vi "SparkFun Motor Driver.vi"() -> ()   [LabVIEW 2016]
uses:
  VIs/uPythonX/uPythonX.xctl
panel:
  in  "Tab Control":T1(tab)=enum."Tacho - interrupt"
  in  "Motors":T2(xcontrol)={"VISA Refnum in"="ASRL23::INSTR", "Python Code"="# In 1    In2    PWM   Out1    Out2    Mode\n#   H       H       H/L       L          L        short break\n#   L        H         H        L          H        CCW\n#   L        H         L        L          H        short break\n#   H        L         H       H          L        CW\n#   H        L         L        L          H       short break\n#   L         L         L        L          L        Stop\n\n# STBY must be high\n\nfrom pyb import Pin, Timer\n\nA_PWM = Pin('W29') # W29 has TIM2, CH2\nAIn2 = Pin('W22', Pin.OUT)\nAIn1 = Pin('W16',Pin.OUT)\nStdby = Pin('W24',Pin.OUT)\n\nBIn1 = Pin('Y12', Pin.OUT)\nBIn2 = Pin('W32',Pin.OUT)\nB_PWM = Pin('Y11') #  TIM8, CH2\n\ntimA = Timer(2, freq=1000)\ntimB = Timer(8, freq=1000)\n\nSpeedA = -50\nSpeedB = 50\n\nStdby.value(0)  #turn motors off until reset\n\nif (SpeedA < 0):\n     AIn1.value(255)\n     AIn2.value(0)\n     SpeedA = - SpeedA\nelse:\n     AIn1.value(0)\n     AIn2.value(255)\n\nif (SpeedB < 0):\n     BIn1.value(255)\n     BIn2.value(0)\n     SpeedB = - SpeedB\nelse:\n     BIn1.value(0)\n     BIn2.value(255)\n\nchA = timA.channel(2, Timer.PWM, pin= A_PWM)\nchA.pulse_width_percent(SpeedA)\nchB = timB.channel(2, Timer.PWM, pin= B_PWM)\nchB.pulse_width_percent(SpeedB)\n\nStdby.value(255)  #everything is ready - reset motors\n"}
  in  "Tacho":T2(xcontrol)={"VISA Refnum in"="ASRL23::INSTR", "Python Code"="# Old |      New Value\n#        |    0    1   2   3\n#   0   |    0   -1  1   X\n#   1   |    1    0   X  -1\n#   2   |   -1   X   0   1\n#   3   |    X    1  -1  0\n\n\n# From https://cdn.sparkfun.com/datasheets/Robotics/How%20to%20use%20a%20quadrature%20encoder.pdf\n\nfrom pyb import Pin\nimport array\nimport utime\n\nM1_New = 0\nM1_EncA = Pin('Y1', Pin.IN, pull = Pin.PULL_UP)\nM1_EncB = Pin('Y2', Pin.IN, pull = Pin.PULL_UP)\n\nM1_Matrix = array.array('l',[0,-1,1,2,1,0,2,-1,-1,2,0,1,2,1,-1,0])\n\n#To read the array my index is: Old * 4 + New So my code reads like this:\nwhile True:\n     M1_Old = M1_New\n     M1_New = M1_EncA.value()  * 2 + M1_EncB.value()\n     Out = M1_Matrix [M1_Old * 4 + M1_New]\n     print('Old: %2d   New: %2d    Out %2d' % (M1_Old, M1_New, Out))\n     utime.sleep(0.01)\n"}
  in  "Tacho 2":T2(xcontrol)={"VISA Refnum in"="ASRL23::INSTR", "Python Code"="# From https://github.com/peterhinch/micropython-samples/blob/master/encoders/encoder.py\n\nfrom pyb import Pin\nimport utime\n\nclass Encoder(object):\n    def __init__(self, pin_x, pin_y, reverse, scale):\n        self.reverse = reverse\n        self.scale = scale\n        self.forward = True\n        self.pin_x = pin_x\n        self.pin_y = pin_y\n        self._pos = 0\n        self.x_interrupt = pyb.ExtInt(pin_x, pyb.ExtInt.IRQ_RISING_FALLING, pyb.Pin.PULL_NONE, self.x_callback)\n        self.y_interrupt = pyb.ExtInt(pin_y, pyb.ExtInt.IRQ_RISING_FALLING, pyb.Pin.PULL_NONE, self.y_callback)\n\n    def x_callback(self, line):\n        self.forward = self.pin_x.value() ^ self.pin_y.value() ^ self.reverse\n        self._pos += 1 if self.forward else -1\n\n    def y_callback(self, line):\n        self.forward = self.pin_x.value() ^ self.pin_y.value() ^ self.reverse ^ 1\n        self._pos += 1 if self.forward else -1\n\n    @property\n    def position(self):\n        return self._pos*self.scale\n\n    def reset(self):\n        self._pos = 0\n\npin1 = Pin('Y4', Pin.IN)\npin2 = Pin('Y3', Pin.IN)\n\ne=Encoder(pin1,pin2,False,0.5)\ne.reset()\nwhile True:\n     e.position\n     utime.sleep(1)"}
  in  "PyBoard":T2(xcontrol)={"VISA Refnum in"="ASRL23::INSTR", "Python Code"="import time,pyb\n\nuart = pyb. UART(3,9600, bits=8, parity=None, stop=1)\n\nwhile(True):\n    time.sleep_ms(100)\n    size = uart.any()\n    if (size > 0):\n        string = uart.read(size)\n        data = int(string[-1])\n        print('Data: %3d' % (data))\n\n\n"}
  in  "Camera":T2(xcontrol)={"VISA Refnum in"="ASRL12::INSTR", "Python Code"="# Show intensity mean\n\nimport sensor, image, time\nimport pyb\n\nclock = time.clock()\nsensor.reset()\nsensor.set_pixformat(sensor.RGB565)\nsensor.set_framesize(sensor.QVGA)\nsensor.skip_frames(time = 2000)\nsensor.set_auto_gain(True)\nsensor.set_auto_whitebal(True) \n\n\nuart = pyb.UART(3,9600, bits=8, parity=None, stop=1)\n\nprint('Starting...')\nwhile(True):\n    clock.tick()\n    img = sensor.snapshot()\n    data = img.statistics()[0]\n    end = uart.write(chr(data))\n"}
  in  "Test":T2(xcontrol)={"VISA Refnum in"="ASRL23::INSTR", "Python Code"="# from https://docs.micropython.org/en/latest/reference/isr_rules.html\n\nimport pyb, micropython\nmicropython.alloc_emergency_exception_buf(100)  # this makes verbose debugging\n\n\nclass LightShow(object):\n    def __init__(self,timer, led):\n        self.led = led\n        timer.callback(self.ToggleIt)\n    def ToggleIt (self,line):\n        self.led.toggle()\n\ntimer1 = pyb.Timer(4, freq=1)\ntimer2 = pyb.Timer(2, freq=0.8)\nled1 =  pyb.LED(1)\nled2 = pyb.LED(2)\n\nred = LightShow(timer1,led1)\ngreen = LightShow(timer2,led2 )\n\n\n# you need to hit Ctrl D to stop the interrupts\n"}
  # "Motor1"
  # "Motor2"
  # "Tx"
  # "Rx"
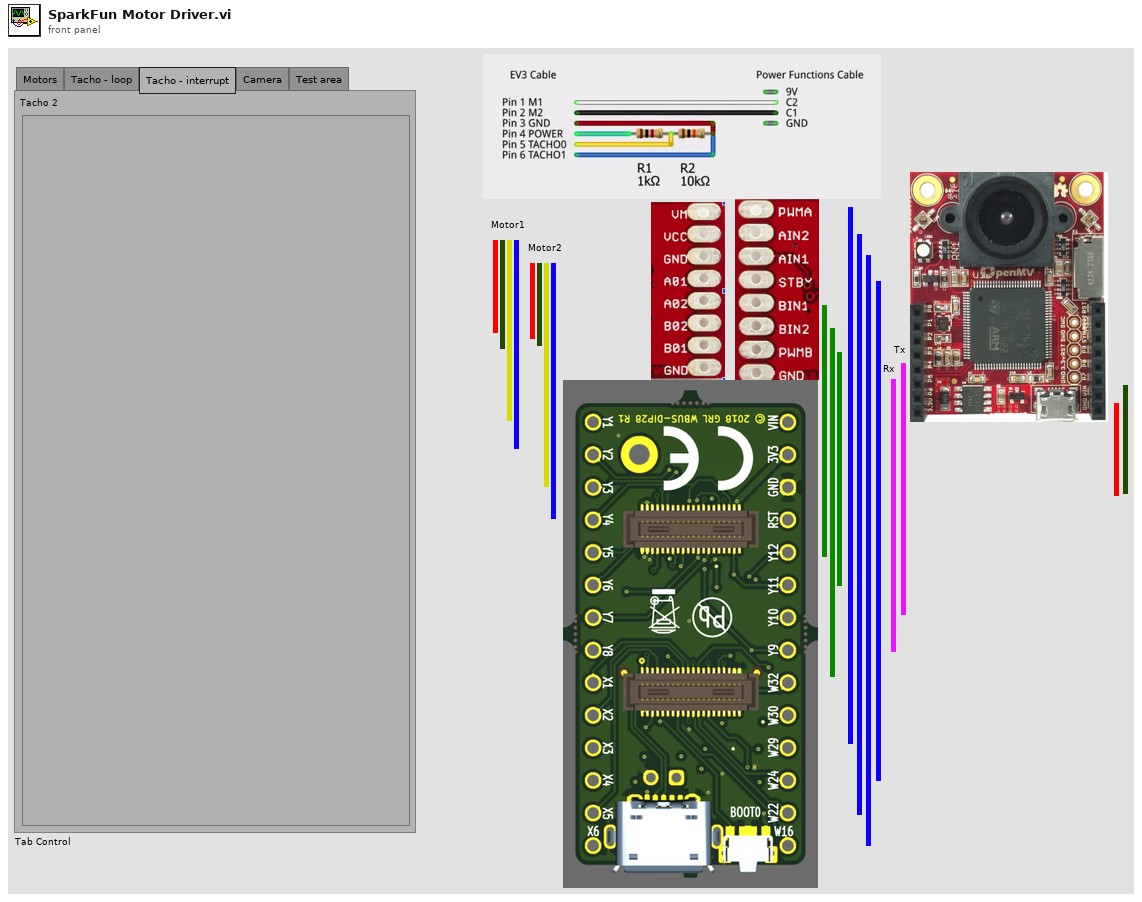
[diagram p1: front panel]
types:
  T1 = enum32{"Motors", "Tacho - loop", "Tacho - interrupt", "Camera", "Test area"}
  T2 = cluster{"VISA Refnum in":refnum<visa-resource-name>, "Python Code":string}
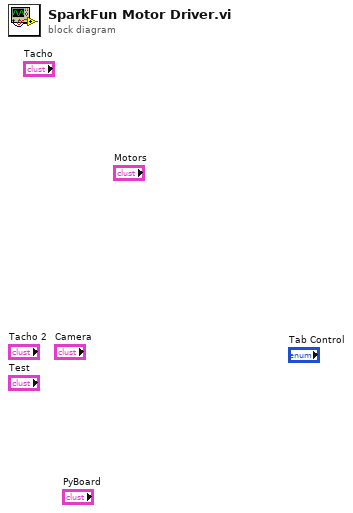
[diagram p0: block diagram]
diagram:
